vi "buildURL.vi"(10 "DataName":string, 11 "parentURL":string) -> (3 "DataURL":string)   [LabVIEW 2017, in "TagDB.lvlib"]
uses:
  TagDB.lvlib
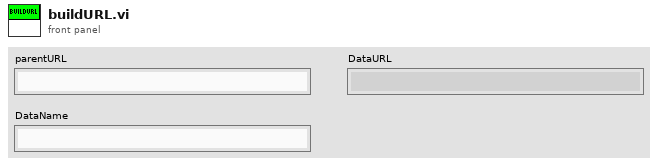
[diagram p1: front panel]
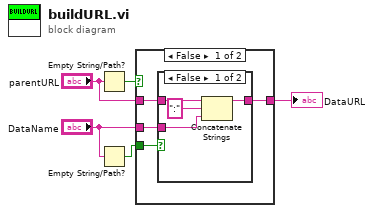
[diagram p0: block diagram]
diagram:
  n1 = Empty String/Path?(string/path="parentURL") -> (empty?=w4:bool)
  n2 = Empty String/Path?(string/path="DataName") -> (empty?=w1:bool)
  n3 = case shown="False" w4 {
    tunnel: "DataName" -> [w9 w15]
    tunnel: [w8 w15] -> w5
    tunnel: "parentURL" -> [w7 _]
    tunnel: w1 -> [w6 _]
    frame False {
      n4 = case shown="False" w6 {
        tunnel: w9 -> [w13 _]
        tunnel: [w12 w14] -> w8
        tunnel: w7 -> [w10 w14]
        frame False {
          n5 = Concatenate Strings(w10, ":" ("string"), w13) -> (w12:string)
        }
        frame True {
        }
      }
    }
    frame True {
    }
  }
  "DataURL" <- w5
